vi "Keep IE in Memory.vi"   [LabVIEW 2021]
uses:
  <vilib>/LabVIEW Icon API/lv_icon/lv_icon.lvlib
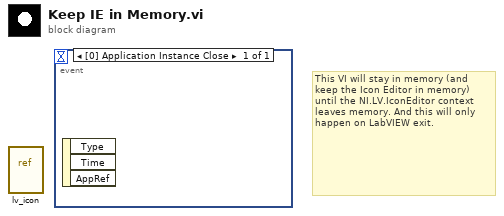
[diagram p0: block diagram]
diagram:
  # "This VI will stay in memory (and keep the Icon Editor in memory) until the NI.LV.IconEditor context leaves memory. And this will only happen on LabVIEW exit."
  n1 = vi-ref <resource>:"lv_icon.vi"() -> ()  [unwired: 1 out]
  n2 = event shown="[0] Application Instance Close" {
    selector: _ -> [_]
    dyn-events: _ -> [_]
    timeout: _ -> [_]
    event Application Instance Close {
      n3 = event-data() -> ()  [unwired: 4 out]
    }
  }
